vi "test_CCDGetConfig.vi"(8 "error in":errorcluster) -> (0 "error out":errorcluster)   [LabVIEW 2023]
uses:
  Classes/CCD/Gain.ctl
  Classes/CCD/Signal.ctl
  Classes/CCD/Event.ctl
  Classes/CCD/Type.ctl
  Classes/CCD/Speed.ctl
  Classes/CCD/Trigger.ctl
  Classes/CCD/GetConfig.ctl
  Classes/CCD/SupportedFeatures.ctl
  Classes/CCD/CCD.lvclass
  C:/Projects/Horiba/horiba-labview-sdk/Source/Classes/GenericDevice/GenericDevice.lvclass
  <vilib>/addons/_JKI Toolkits/Caraya/classes/Assert/Assert Equal Value_Variant.vi
  <vilib>/addons/_JKI Toolkits/Caraya/classes/Assert/Assert Not Error.vi
  <vilib>/addons/_JKI Toolkits/Caraya/classes/Test/Test.lvclass
  <vilib>/addons/_JKI Toolkits/Caraya/classes/Assert/Assert.lvclass
  C:/Projects/Horiba/horiba-labview-sdk/Source/Classes/CCD/CCD.lvclass
panel:
  out "config-text pairs":string[][](array[string])
  out "config-JSON pairs":string[][](array[string])
  out "config-JSON string":string
  # "Connector Pane"
  # "Locals"
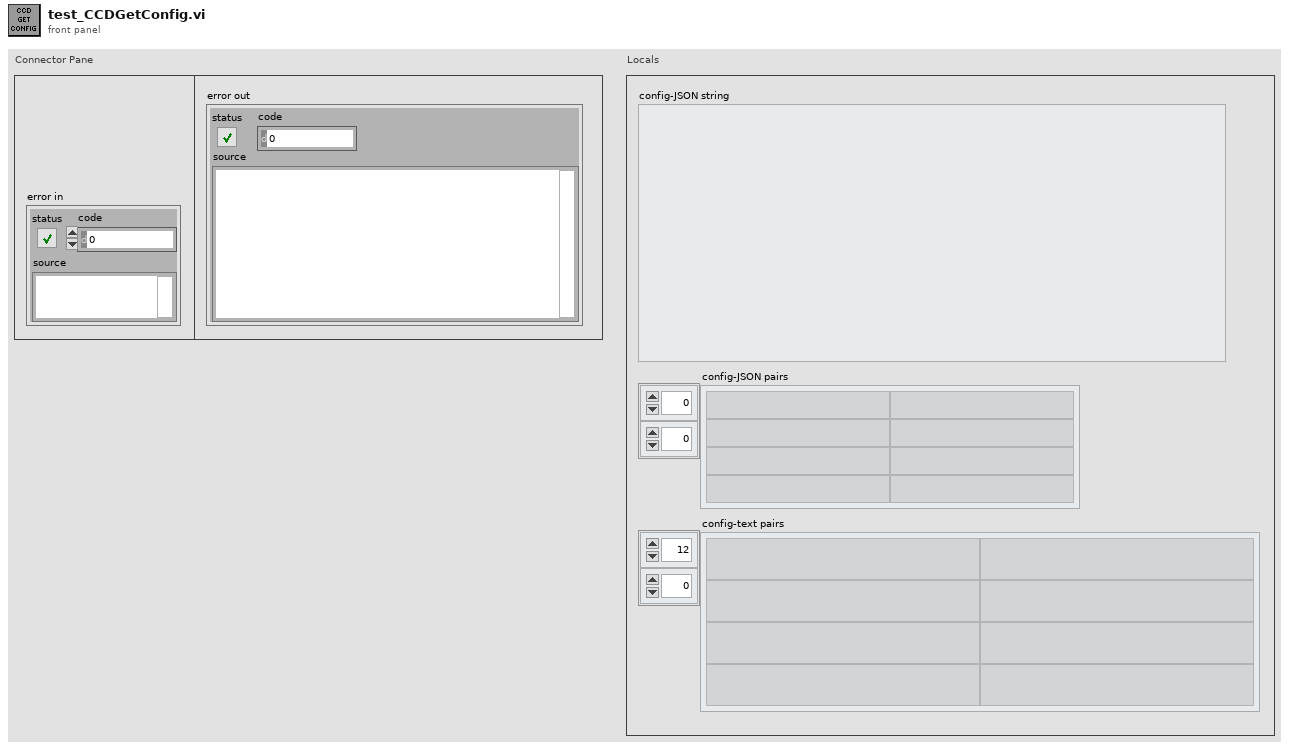
[diagram p1: front panel]
types:
  T1 = typedef "CCD.lvclass/GetConfig.ctl" = cluster{"centerWavelength":dbl, "chipHSpacing":dbl, "chipHeight":dbl, "chipName":string, "chipSerialNumber":string, "chipVSpacing":dbl, "chipWidth":dbl, "deviceType":string, "fitParameters":dbl[], "gains":T2[], "hardwareAvgAvailable":bool, "lineScan":bool, "productId":string, "serialNumber":string, "signals":T3[], "speeds":T6[], "supportedFeatures":T7, "triggers":T8[], "version":string}
  T2 = typedef "CCD.lvclass/Gain.ctl" = cluster{"info":string, "token":i32}
  T3 = typedef "CCD.lvclass/Signal.ctl" = cluster{"events":T4[], "name":string, "token":i32}
  T4 = typedef "CCD.lvclass/Event.ctl" = cluster{"name":string, "token":i32, "types":T5[]}
  T5 = typedef "CCD.lvclass/Type.ctl" = cluster{"name":string, "token":i32}
  T6 = typedef "CCD.lvclass/Speed.ctl" = cluster{"info":string, "token":i32}
  T7 = typedef "CCD.lvclass/SupportedFeatures.ctl" = cluster{"cf_3PositionSlit":bool, "cf_CMOSOffsetCorrection":bool, "cf_Cleaning":bool, "cf_DSP":bool, "cf_DSPBin2X":bool, "cf_DelayAfterTrigger":bool, "cf_Delays":bool, "cf_EMCCD":bool, "cf_EShutter":bool, "cf_HDR":bool, "cf_Image":bool, "cf_MemorySlots":bool, "cf_Metadata":bool, "cf_MultipleExposeTimes":bool, "cf_MultipleSensors":bool, "cf_PulseSummation":bool, "cf_ROIs":bool, "cf_Signals":bool, "cf_Spectra":bool, "cf_TriggerQualifier":bool, "cf_Triggers":bool}
  T8 = typedef "CCD.lvclass/Trigger.ctl" = cluster{"events":T4[], "name":string, "token":i32}
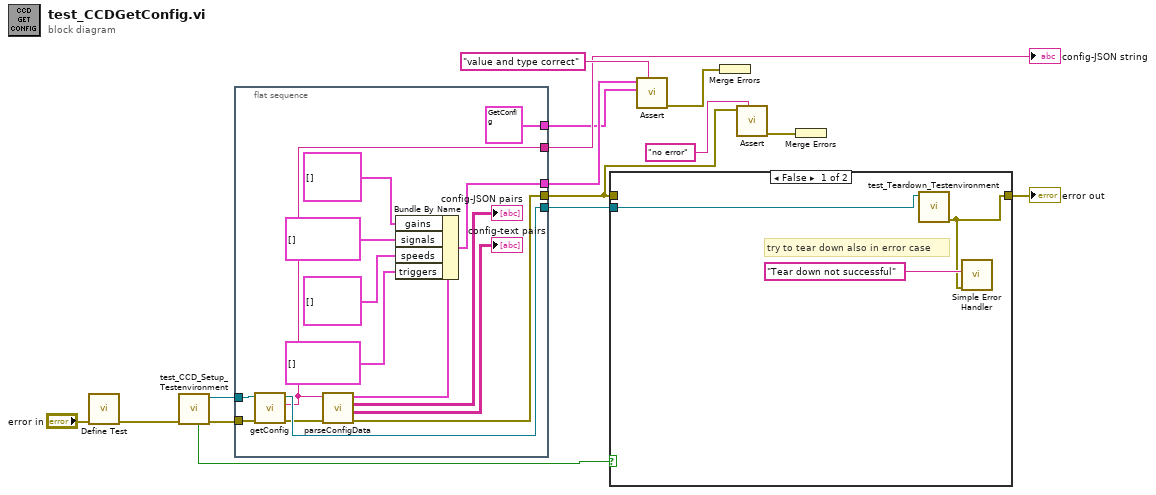
[diagram p0: block diagram]
diagram:
  n1 = call <vilib>:"Define Test.vi"("error in (no error)"="error in") -> ("error out"=w2:errorcluster)  [unwired: 9 in, 1 out]
  n2 = call "test_CCD_Setup_Testenvironment.vi"("error in"=w2) -> ("error out"=w4:errorcluster, "CCD out"=w3:refnum<class "CCD.lvclass">, "Module Was Already Running?"=w1:bool)  [unwired: 7 in, 1 out]
  n3 = flat-sequence {
    tunnel: [w27] -> w13
    tunnel: w4 -> [w30]
    tunnel: w3 -> [w29]
    tunnel: [w25] -> w9
    tunnel: [w28] -> w8
    tunnel: [w21] -> w6
    tunnel: [T1 {"centerWavelength"=0.0, "chipHSpacing"=260.0, "chipHeight"=256.0, "chipName"="CCD30-11-1-275", "chipSerialNumber"="20091-22-21", "chipVSpacing"=260.0, "chipWidth"=1024.0, "deviceType"="HORIBA Syncerity", "fitParameters"=[0.0, 1.0, 0.0, 0.0, 0.0], "gains"=[], "hardwareAvgAvailable"=FALSE, "lineScan"=FALSE, "productId"="13", "serialNumber"="Camera SN:  2244", "signals"=[], "speeds"=[], "supportedFeatures"={"cf_3PositionSlit"=FALSE, "cf_CMOSOffsetCorrection"=FALSE, "cf_Cleaning"=TRUE, "cf_DSP"=FALSE, "cf_DSPBin2X"=FALSE, "cf_DelayAfterTrigger"=FALSE, "cf_Delays"=FALSE, "cf_EMCCD"=FALSE, "cf_EShutter"=FALSE, "cf_HDR"=FALSE, "cf_Image"=TRUE, "cf_MemorySlots"=TRUE, "cf_Metadata"=FALSE, "cf_MultipleExposeTimes"=FALSE, "cf_MultipleSensors"=FALSE, "cf_PulseSummation"=FALSE, "cf_ROIs"=TRUE, "cf_Signals"=TRUE, "cf_Spectra"=TRUE, "cf_TriggerQualifier"=FALSE, "cf_Triggers"=TRUE}, "triggers"=[], "version"="Syncerity Ver 1.001.7.1"} ("output cluster")] -> w5
    frame #0 {
      n4 = call "getConfig.vi"("error in (no error)"=w30, "CCD in"=w29) -> ("error out"=w26:errorcluster, "config-JSON string"=w27:string, "CCD out"=w28:refnum<class "CCD.lvclass">)  [unwired: 7 in]
      n5 = call "parseConfigData.vi"("error in (no error)"=w26, "results-JSON string"=w27) -> ("error out"=w25:errorcluster, "config-text pairs"=→"config-text pairs":string[][], "config-JSON pairs"=→"config-JSON pairs":string[][], "config data"=w22:T1)  [unwired: 6 in]
      n6 = Bundle By Name(cluster=w22, "gains"=T2[] [], "signals"=T3[] [], "speeds"=T6[] [], "triggers"=T8[] []) -> (w21:T1)
    }
  }
  n7 = case shown="False" w1 {
    tunnel: w8 -> [w32 _]
    tunnel: [w31 w34] -> w7
    tunnel: w9 -> [_ w34]
    frame False {
      # "try to tear down also in error case"
      n8 = call "test_Teardown_Testenvironment.vi"("GenericDevice.lvclass"=w32) -> ("error out"=w31:errorcluster)  [unwired: 9 in, 1 out]
      n9 = call <vilib>:"Simple Error Handler.vi"("error source (\" \")"="Tear down not successful" ("error source (\" \")"), "error in (no error)"=w31) -> ()  [unwired: 3 in, 5 out]
    }
    frame True {
    }
  }
  "error out" <- w7
  n10 = call-poly <vilib>:"Assert.vi"("Label"="value and type correct" ("Label (VI Title)"), "Y"=w5, "X"=w6) -> ("error out"=w14:errorcluster)  [unwired: 7 in, 1 out]
  n11 = Merge Errors(w14) -> ()  [unwired: 1 out]
  n12 = call-poly <vilib>:"Assert.vi"("Label"="no error" ("Label (VI Title)"), "Not Error?"=w9) -> ("error out"=w10:errorcluster)  [unwired: 8 in, 1 out]
  n13 = Merge Errors(w10) -> ()  [unwired: 1 out]
  "config-JSON string" <- w13
